vi "Initialize Sink.vi"(11 "Text File Sink in":refnum<class "Text File Sink.lvclass">) -> (0 "error out":errorcluster, 3 "Text File Sink out":refnum<class "Text File Sink.lvclass">)   [LabVIEW 2017, in "Text File Sink.lvclass"]
uses:
  Text File Sink.lvclass
  Text File Sink.lvclass/Text File Sink.ctl
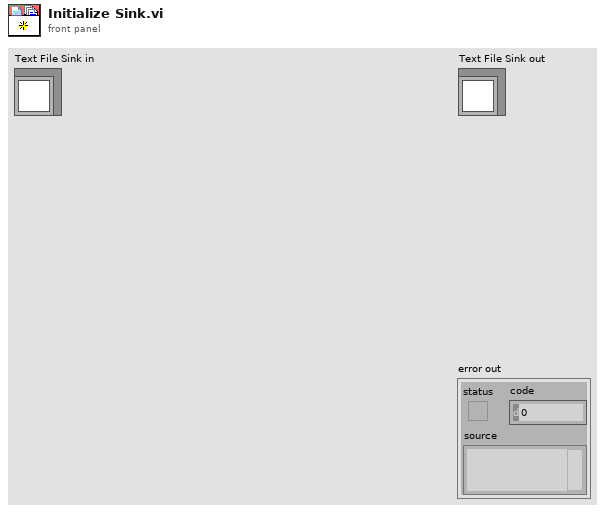
[diagram p1: front panel]
types:
  T1 = typedef "LVDateTimeRec.ctl" = cluster{"fractional second":dbl, "second":i32, "minute":i32, "hour":i32, "day of month":i32, "month":i32, "year":i32, "day of week":i32, "day of year":i32, "DST":i32}
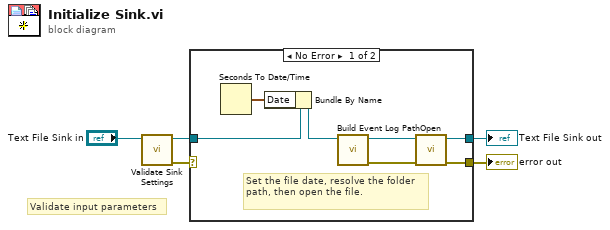
[diagram p0: block diagram]
diagram:
  # "Validate input parameters"
  n1 = call "Validate Sink Settings.vi"("Text File Sink in"="Text File Sink in") -> ("error out"=w1:errorcluster, "Text File Sink out"=w2:refnum<class "Text File Sink.lvclass">)  [unwired: 9 in]
  n2 = case shown="No Error" w1 {
    selector: w1 -> [_ w13]
    tunnel: [w12 w14] -> w5
    tunnel: [w9 w13] -> w4
    tunnel: w2 -> [w6 w14]
    frame No Error {
      # "Set the file date, resolve the folder path, then open the file."
      n3 = Seconds To Date/Time() -> (date time rec=w7:T1)  [unwired: 2 in]
      n4 = Bundle By Name(cluster=w6, "Date"=w7) -> (w8:refnum<class "Text File Sink.lvclass">)
      n5 = call "Build Event Log Path.vi"("Text File Sink in"=w8) -> ("error out"=w10:errorcluster, "Text File Sink out"=w11:refnum<class "Text File Sink.lvclass">)  [unwired: 9 in]
      n6 = call "Open.vi"("error in (no error)"=w10, "Text File Sink in"=w11) -> ("error out"=w9:errorcluster, "Text File Sink out"=w12:refnum<class "Text File Sink.lvclass">)  [unwired: 8 in]
    }
    frame Error {
      # "One or more input parameters is invalid - pass error back to user and don't initialize sink"
    }
  }
  "error out" <- w4
  "Text File Sink out" <- w5
